vi "StageA_00_BandPass.vi"(9 "s_axis_data_tdata":fxp<+/-,16,1>, 10 "s_axis_data_tvalid":bool) -> (1 "m_axis_data_tdata":fxp<+/-,24,2>, 2 "m_axis_data_tvalid":bool, 3 "s_axis_data_tready":bool)   [LabVIEW 2018]
uses:
  <vilib>/rvi/XilinxIP/XIPIN_XNode/niFpgaXIPIN.xnode
  DigitalFilterDesign/FIR_Filter_Configuration/FIR Compiler/xsim.dir/FIR_Compiler_3CE652926F5B43F18022D1349C670FA0/xsimk_3CE652926F5B43F18022D1349C670FA0.dll
  <vilib>/rvi/IPIntegrationNode/IPINode_Xnode/niFpgaIPINode.xnode
  <vilib>/rvi/IPIntegrationNode/IPINode_Typedef/niFpgaIPINodeSupportedFamilies.ctl
  <vilib>/rvi/IPIntegrationNode/IPINode_Utilities/niFpgaIPINodeSimCore.vi
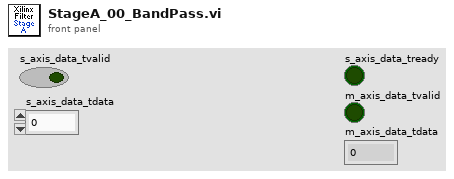
[diagram p1: front panel]
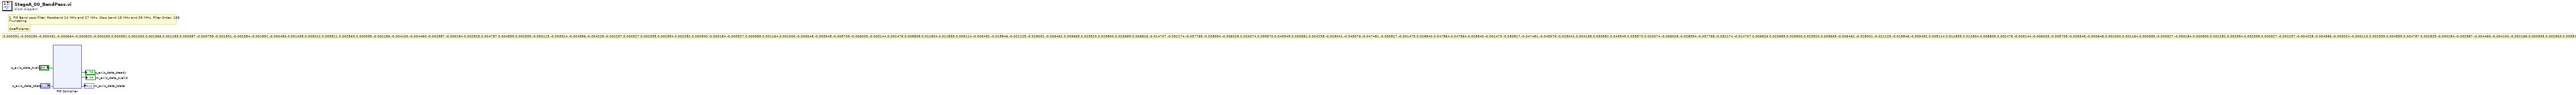
[diagram p0: block diagram]
diagram:
  # "0.000391,-0.000280,-0.000491,-0.000664,-0.000620,-0.000263,0.000351,0.001000,0.001366,0.001183,0.000387,-0.000799,-0.001901,-0.002384,-0.001891,-0.000456,0.001438,0.003012,0.003511,0.002563,0.000395,-0.002186,-0.004100,-0.004460,-0.002987,-0.000184,0.002829,0.004787,0.004839,0.002939,-0.000113,-0.003024,-0.004586,-0.004228,-0.002257,0.000327,0.002338,0.002994,0.002282,0.000900,-0.000184,-0.000327,0.000385,0.001164,0.001000,-0.000648,-0.003348,-0.005709,-0.006003,-0.003144,0.002478,0.008805,0.012804,0.011835,0.005114,-0.005492,-0.015846,-0.021125,-0.018001,-0.006462,0.009665,0.023920,0.029800,0.023689,0.006826,-0.014707,-0.032174,-0.037765,-0.028094,-0.006028,0.020074,0.039570,0.043949,0.030581,0.004138,-0.025041,-0.045076,-0.047481,-0.030817,-0.001473,0.028840,0.047864,0.047864,0.028840,-0.001473,-0.030817,-0.047481,-0.045076,-0.025041,0.004138,0.030581,0.043949,0.039570,0.020074,-0.006028,-0.028094,-0.037765,-0.032174,-0.014707,0.006826,0.023689,0.029800,0.023920,0.009665,-0.006462,-0.018001,-0.021125,-0.015846,-0.005492,0.005114,0.011835,0.012804,0.008805,0.002478,-0.003144,-0.006003,-0.005709,-0.003348,-0.000648,0.001000,0.001164,0.000385,-0.000327,-0.000184,0.000900,0.002282,0.002994,0.002338,0.000327,-0.002257,-0.004228,-0.004586,-0.003024,-0.000113,0.002939,0.004839,0.004787,0.002829,-0.000184,-0.002987,-0.004460,-0.004100,-0.002186,0.000395,0.002563,0.003511,0.003012,0.001438,-0.000456,-0.001891,-0.002384,-0.001901,-0.000799,0.000387,0.001183,0.001366,0.001000,0.000351,-0.000263,-0.000620,-0.000664,-0.000491,-0.000280,0.000391"
  # "Coefficients:"
  # "1.\tFIR Band pass filter. Passband 24 MHz and 27 MHz. Stop band 19 MHz and 33 MHz. Filter Order: 138 \nTruncating"
  n1 = xnode ("FIR Compiler")("s_axis_data_tvalid"="s_axis_data_tvalid", "s_axis_data_tdata"="s_axis_data_tdata") -> ("s_axis_data_tready"=→"s_axis_data_tready":bool, "m_axis_data_tvalid"=→"m_axis_data_tvalid":bool, "m_axis_data_tdata"=→"m_axis_data_tdata":fxp<+/-,24,2>)
